vi "Create AI with Conversion Filter Channel.vi"(6 "index":i32, 7 "conversion time":T1, 8 "error in":errorcluster, 9 "default value":dbl, 10 "name":string, 11 "AI with conversion filter channel in":refnum<class "AI with Conversion Filter Channel.lvclass">) -> (0 "error out":errorcluster, 3 "AI with conversion filter channel out":refnum<class "AI with Conversion Filter Channel.lvclass">)   [LabVIEW 2017, in "Scan Engine Scripting.lvlib" / "AI with Conversion Filter Channel.lvclass"]
uses:
  AI with Conversion Filter Channel.lvclass
  Conversion Time.ctl
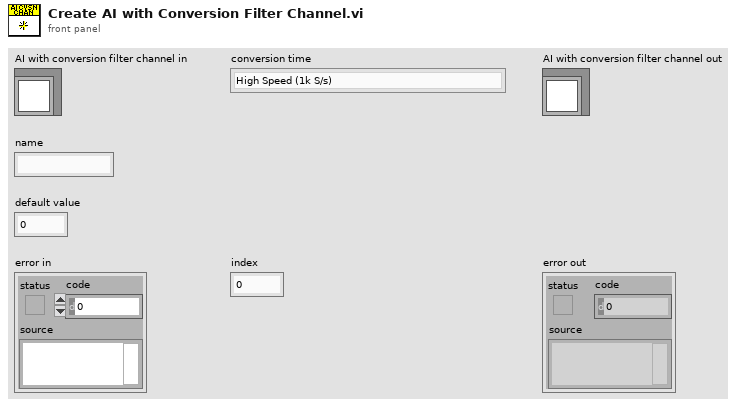
[diagram p1: front panel]
types:
  T1 = typedef "Scan Engine Scripting.lvlib/AI with Conversion Filter Channel.lvclass/Conversion Time.ctl" = enum16{"High Speed (1k S/s)", "Medium Speed (100 S/s)", "Medium Resolution (50/60 Hz Rejection - 12 S/s)", "High Resolution (50/60 Hz Rejection - 2 S/s)"}
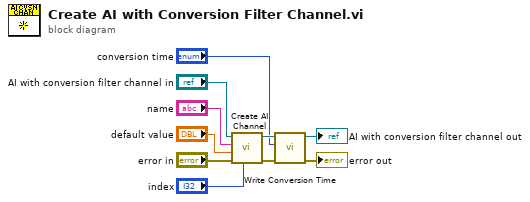
[diagram p0: block diagram]
diagram:
  n1 = call-dynamic "Create AI Channel.vi"("index"="index", "error in"="error in", "default value"="default value", "name"="name", "AI channel in"="AI with conversion filter channel in") -> ("error out"=w5:errorcluster, "AI channel out"=w6:refnum<class "AI with Conversion Filter Channel.lvclass">)  [unwired: 5 in]
  n2 = call-dynamic "Write Conversion Time.vi"("error in"=w5, "conversion time"="conversion time", "AI with conversion filter channel in"=w6) -> ("error out"=→"error out":errorcluster, "AI with conversion filter channel out"=→"AI with conversion filter channel out":refnum<class "AI with Conversion Filter Channel.lvclass">)  [unwired: 7 in]
